vi "main.vi"() -> ()   [LabVIEW 2018]
panel:
  in  "Tab Control":T1(tab)
  in  "#1":dbl
  in  "#2":dbl
  out "Average":dbl
  in  "hits":dbl
  in  "strikeouts":dbl
  in  "Base on \nError":dbl
  in  "Other \nOuts":dbl
  out "batting\naverage":dbl
  in  "Current\nmonth":dbl
  in  "current\nday":dbl
  in  "current\nyear":dbl
  in  "birth\nmonth":dbl
  in  "birth\nday":dbl
  in  "birth\nyear":dbl
  out "age":dbl
  in  "weight\n(lbs)":dbl
  in  "height\n(inches)":dbl
  out "under\nweight":bool
  out "healthy":bool
  out "over\nweight":bool
  out "obese":bool
  out "under\nweight 2":bool
  out "healthy 2":bool
  out "over\nweight 2":bool
  out "obese 2":bool
  in  "stop":bool
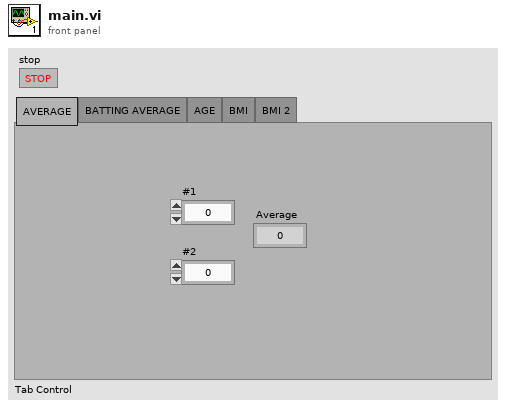
[diagram p1: front panel]
types:
  T1 = enum32{"AVERAGE", "BATTING AVERAGE", "AGE", "BMI", "BMI 2"}
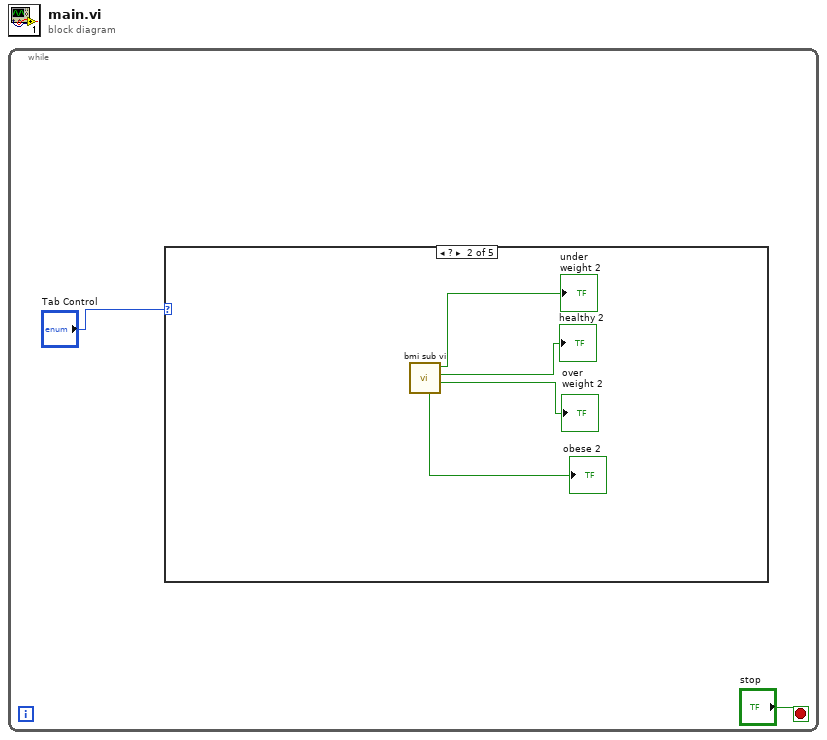
[diagram p0: block diagram]
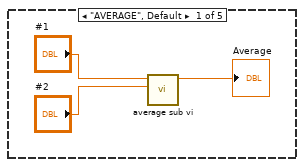
[diagram p2: hidden frame]
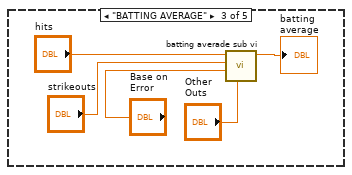
[diagram p3: hidden frame]
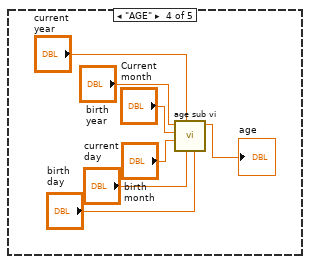
[diagram p4: hidden frame]
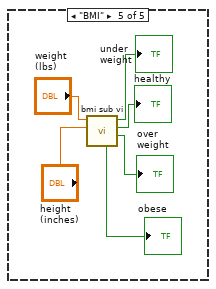
[diagram p5: hidden frame]
diagram:
  n1 = while {
    stop <- "stop" stop-if-true
    n2 = case "Tab Control" {
      frame "AVERAGE", Default {
        n3 = call "average sub vi.vi"("Numeric 2"="#2", "Numeric"="#1") -> ("Numeric 3"=→"Average":dbl)  [unwired: 9 in]
      }
      frame ? {
        n4 = call "bmi sub vi.vi"() -> ("over\nweight"=→"over\nweight 2":bool, "healthy"=→"healthy 2":bool, "under\nweight"=→"under\nweight 2":bool, "obese"=→"obese 2":bool)  [unwired: 8 in]
      }
      frame "BATTING AVERAGE" {
        n5 = call "batting averade sub vi.vi"("Other \nOuts"="Other \nOuts", "Base on \nError"="Base on \nError", "strikeouts"="strikeouts", "hits"="hits") -> ("batting\naverage"=→"batting\naverage":dbl)  [unwired: 7 in]
      }
      frame "AGE" {
        n6 = call "age sub vi.vi"("birth\nday"="birth\nday", "current\nday"="current\nday", "current\nyear"="current\nyear", "birth\nmonth"="birth\nmonth", "Current\nmonth"="Current\nmonth", "birth\nyear"="birth\nyear") -> ("age"=→"age":dbl)  [unwired: 5 in]
      }
      frame "BMI" {
        n7 = call "bmi sub vi.vi"("height\n(inches)"="height\n(inches)", "weight\n(lbs)"="weight\n(lbs)") -> ("over\nweight"=→"over\nweight":bool, "healthy"=→"healthy":bool, "under\nweight"=→"under\nweight":bool, "obese"=→"obese":bool)  [unwired: 6 in]
      }
    }
  }
